vi "Set Pump State.vi"(8 "error in (no error)":cluster{"状态":bool, "代码":i32, "源":string} caption="错误输入（无错误）", 10 "泵状态":bool, 11 "仿真蒸发冷却器输入":refnum<class "Simulated Evaporative Cooler.lvclass">) -> (0 "error out":cluster{"状态":bool, "代码":i32, "源":string} caption="错误输出")   [LabVIEW 2013, in "Simulated Evaporative Cooler.lvclass"]
uses:
  Simulated Evaporative Cooler.lvclass
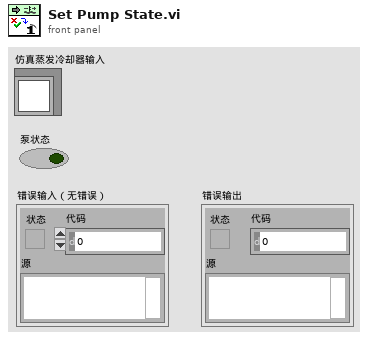
[diagram p1: front panel]
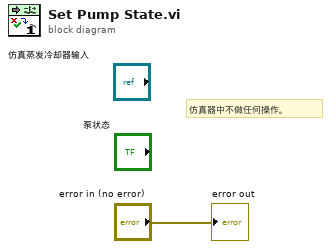
[diagram p0: block diagram]
diagram:
  # "仿真器中不做任何操作。"
  "error out" <- "error in (no error)"
